vi "CMWallTypes.vi"(8 "error in":errorcluster, 10 "Data Type":string, 11 "CMWin":refnum<class "RADEBase.lvclass">) -> (0 "error out":errorcluster, 2 "CMW":string, 3 "CMWout":refnum<class "RADEBase.lvclass">)   [LabVIEW 2014]
uses:
  <userlib>/_RADE/RIO/RADEBase/classes/RADEBase/RADEBase.lvclass
  <userlib>/_RADE/RIO/CMW/classes/CMWSubscribe/CMWSubscribe.lvclass
  <userlib>/_RADE/RIO/CMW/classes/CMWSubscribe/CMWSubscribe.vi
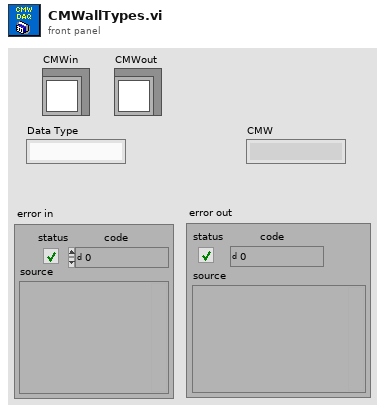
[diagram p1: front panel]
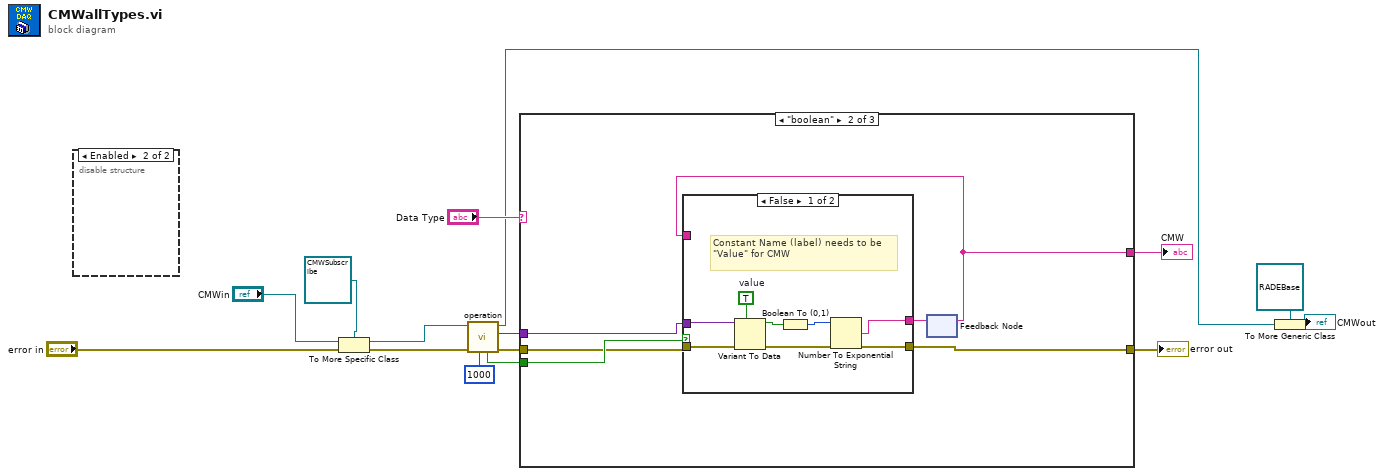
[diagram p0: block diagram]
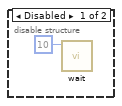
[diagram p2: hidden frame]
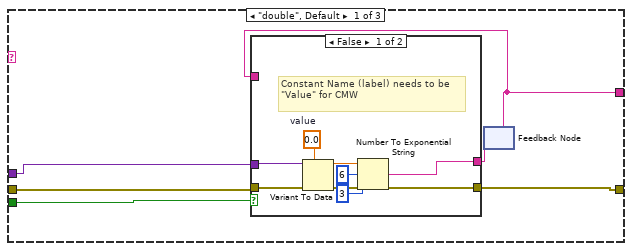
[diagram p3: hidden frame]
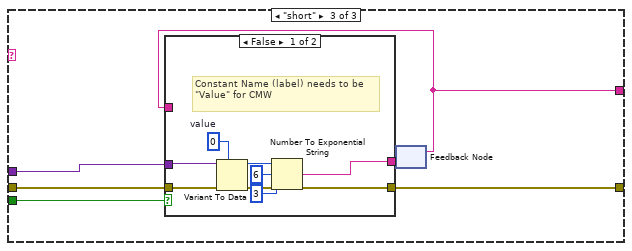
[diagram p6: hidden frame]
diagram:
  n1 = disable-structure shown="Enabled" {
    frame Disabled {
      n2 = call "wait.vi"("milliseconds to wait"=u32 10) -> ()  [unwired: 10 in, 1 out]
    }
    frame Enabled {
    }
  }
  n3 = To More Specific Class(target class=refnum<class "CMWSubscribe.lvclass"> refnum ("Object out"), reference="CMWin", error in="error in") -> (specific class reference=w9:refnum<class "CMWSubscribe.lvclass">, error out=w8:errorcluster)
  n4 = call-poly <userlib>:"operation.vi"("Timeout (10000 ms)"=1000, "error in (no error)"=w8, "Object in"=w9) -> ("error out"=w7:errorcluster, "Data"=w6:variant, "Object out"=w2:refnum<class "CMWSubscribe.lvclass">, "Timeout?"=w5:bool)  [unwired: 4 in, 1 out]
  n5 = case shown="\"boolean\"" "Data Type" {
    tunnel: w7 -> [w18 w36 w52]
    tunnel: [w20 w34 w49] -> w15
    tunnel: [w21 w33 w50] -> w13
    tunnel: w6 -> [w17 w35 w48]
    tunnel: w5 -> [w19 w37 w51]
    frame "double", Default {
      n6 = feedback #1() -> (w21:string)  [unwired: 1 in]
      n7 = case shown="False" w19 {
        tunnel: w18 -> [w30 w32]
        tunnel: [w28 w32] -> w20
        tunnel: w17 -> [w29 _]
        tunnel: [w26 w31] -> w22
        tunnel: w21 -> [_ w31]
        frame False {
          w25 = sgl 0.0  # value
          # "Constant Name (label) needs to be \"Value\" for CMW"
          n8 = Variant To Data(error in=w30, type=w25, Variant=w29) -> (data=w27:sgl, error out=w28:errorcluster)
          n9 = Number To Exponential String(number=w27, precision (6)=i16 3, 3:i16 6 ("width (-)")) -> (E-format string=w26:string)  [unwired: 1 in]
        }
        frame True {
          # "Subscription Timed Out"
        }
      }
      n10 = feedback-in #1(w22) -> ()
    }
    frame "boolean" {
      n11 = feedback #2() -> (w33:string)  [unwired: 1 in]
      n12 = case shown="False" w37 {
        tunnel: w36 -> [w45 w47]
        tunnel: [w43 w47] -> w34
        tunnel: w35 -> [w44 _]
        tunnel: [w42 w46] -> w38
        tunnel: w33 -> [_ w46]
        frame False {
          w41 = TRUE  # value
          # "Constant Name (label) needs to be \"Value\" for CMW"
          n13 = Variant To Data(error in=w45, type=w41, Variant=w44) -> (data=w40:bool, error out=w43:errorcluster)
          n14 = Boolean To (0,1)(Boolean=w40) -> (0, 1=w39:i16)
          n15 = Number To Exponential String(number=w39) -> (E-format string=w42:string)  [unwired: 3 in]
        }
        frame True {
          # "Subscription Timed Out"
        }
      }
      n16 = feedback-in #2(w38) -> ()
    }
    frame "short" {
      n17 = feedback #3() -> (w50:string)  [unwired: 1 in]
      n18 = case shown="False" w51 {
        tunnel: w52 -> [w61 w63]
        tunnel: [w59 w63] -> w49
        tunnel: w48 -> [w60 _]
        tunnel: [w57 w62] -> w53
        tunnel: w50 -> [_ w62]
        frame False {
          w56 = i16 0  # value
          # "Constant Name (label) needs to be \"Value\" for CMW"
          n19 = Variant To Data(error in=w61, type=w56, Variant=w60) -> (data=w58:i16, error out=w59:errorcluster)
          n20 = Number To Exponential String(number=w58, precision (6)=i16 3, 3:i16 6 ("width (-)")) -> (E-format string=w57:string)  [unwired: 1 in]
        }
        frame True {
          # "Subscription Timed Out"
        }
      }
      n21 = feedback-in #3(w53) -> ()
    }
  }
  "error out" <- w15
  "CMW" <- w13
  n22 = To More Generic Class(target class=refnum<class "RADEBase.lvclass"> refnum ("INIT 2"), reference=w2) -> (generic class reference=→"CMWout":refnum<class "RADEBase.lvclass">)
